vi "Move Simulator.vi"(7 "Module Name":string, 8 "error in (no error)":errorcluster, 10 "Target Position":dbl) -> (0 "error out":errorcluster)   [LabVIEW 2019, in "ADLINK Motion Card.lvlib"]
uses:
  ADLINK Motion Card.lvlib
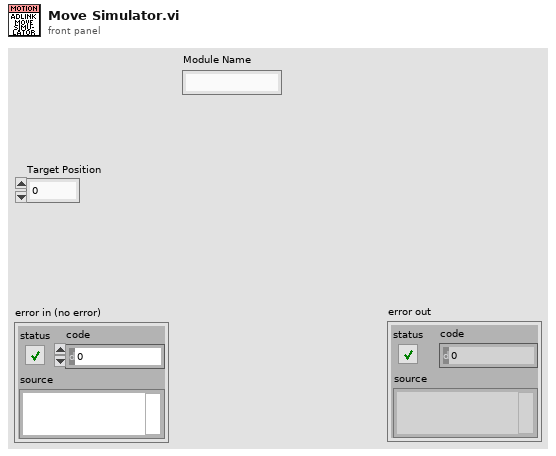
[diagram p1: front panel]
types:
  T1 = typedef "ADLINK Motion Card.lvlib/SEQ Data.ctl" = cluster{"Current Position":dbl, "Target Position":dbl, "Velocity":dbl, "Acceleration":dbl, "Arrived?":bool, "data value reference":refnum<data-value>, "VI Refnum":refnum<vi>}
  T2 = cluster{"Current Position":dbl, "Target Position":dbl, "Velocity":dbl, "Acceleration":dbl, "Arrived?":bool}
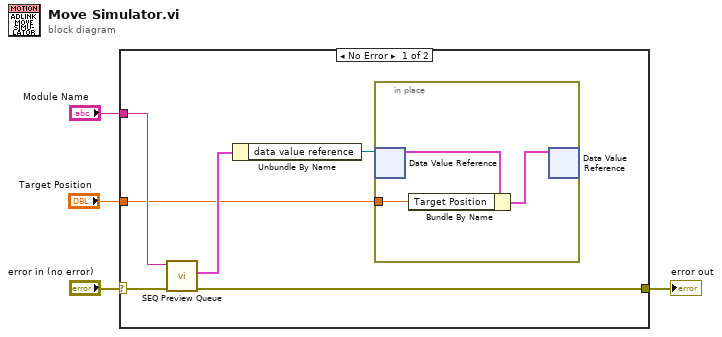
[diagram p0: block diagram]
diagram:
  n1 = case shown="No Error" "error in (no error)" {
    selector: "error in (no error)" -> [w9 w14]
    tunnel: [w5 w14] -> w4
    tunnel: "Module Name" -> [w10 _]
    tunnel: "Target Position" -> [w6 _]
    frame No Error {
      n2 = call "SEQ Preview Queue.vi"("error in (no error)"=w9, "Queue Name"=w10) -> ("error out"=w5:errorcluster, "Setting"=w8:T1)  [unwired: 8 in]
      n3 = Unbundle By Name(w8) -> ("data value reference"=w7:refnum<data-value>)
      n4 = in-place {
        in-place-border: w6 -> [w12]
        n5 = in-place-dvr #1(w7) -> (w13:T2)  [unwired: 1 out]
        n6 = Bundle By Name(cluster=w13, "Target Position"=w12) -> (w11:T2)
        n7 = in-place-dvr #1(w11) -> ()  [unwired: 2 out]
      }
    }
    frame Error {
    }
  }
  "error out" <- w4
